vi "Call Function.vi"(7 "Function Name":string, 8 "Error In":errorcluster, 11 "OPI Ref":refnum<data-value>) -> (0 "Error Out":errorcluster, 3 "OPI Ref":refnum<data-value>)   [LabVIEW 2016, in "OPI.lvclass"]
doc: "Call the python function with predefined arguments. The <b>return value</b> and <b>exception information</b> from the function execution will be captured by the OPI. \n\nThe wired function name should be only the name of the function, <b>without</b> parentheses or arguments.\n\nRead return value with <b>Get Return</b>. The exception will be passed into the error cluster output.\n\n<b>Important</b> - the methods called by OPI should not have infinite loops or other mechanisms blocking execution. This can cause a timeout on the OPI."
uses:
  OPI.lvclass
  OPI.lvclass/OPI.ctl
  <vilib>/Utility/error.llb/Error Cluster From Error Code.vi
  <vilib>/ErrorRing/Error Ring.xnode
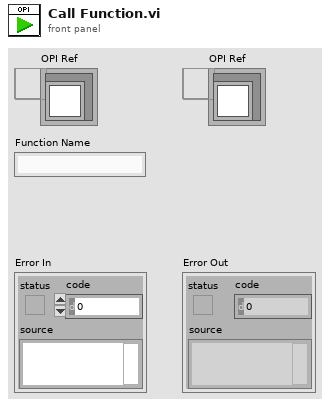
[diagram p1: front panel]
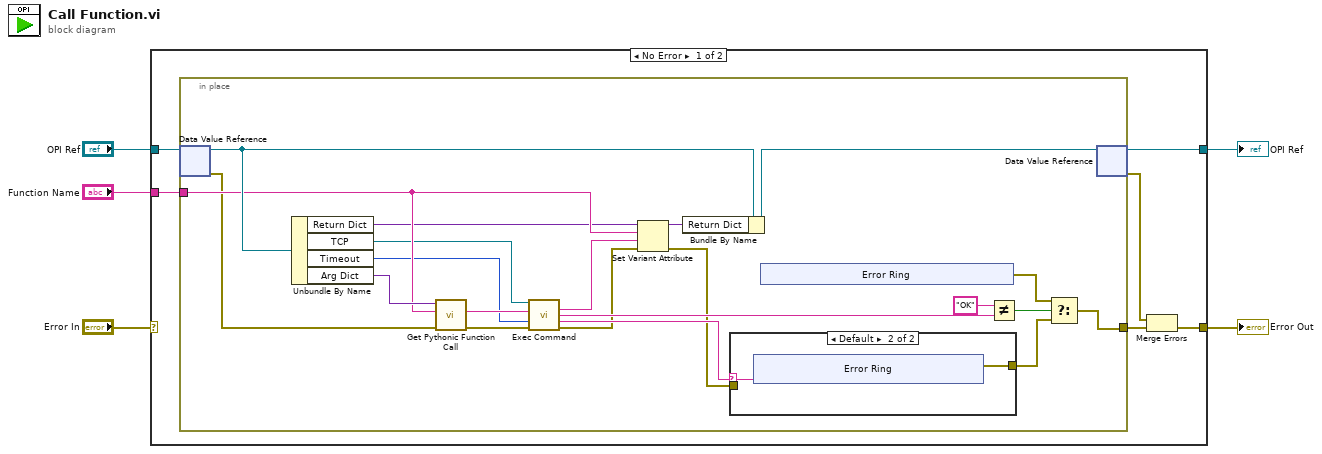
[diagram p0: block diagram]
diagram:
  n1 = case shown="No Error" "Error In" {
    selector: "Error In" -> [_ w48]
    tunnel: [w8 w48] -> w1
    tunnel: "OPI Ref" -> [w11 w49]
    tunnel: [w10 w49] -> w4
    tunnel: "Function Name" -> [w6 _]
    frame No Error {
      n2 = in-place {
        in-place-border: [w28] -> w9
        in-place-border: w6 -> [w18]
        n3 = in-place-dvr #1(w11) -> (w27:refnum<class "OPI.lvclass">, w12:errorcluster)
        n4 = Unbundle By Name(w27) -> ("Return Dict"=w15:variant, "TCP"=w14:refnum<k5>, "Timeout"=w13:i32, "Arg Dict"=w19:variant)
        n5 = call "Get Pythonic Function Call.vi"("Error In"=w12, "Function Name"=w18, "Arg Dict"=w19) -> ("Error Out"=w17:errorcluster, "Function Call"=w16:string)  [unwired: 7 in]
        n6 = call "Exec Command.vi"("TCP In"=w14, "Function Name"=w16, "Timeout"=w13, "Error In"=w17) -> ("Return Value"=w22:string, "OK Ack"=w23:string, "Exception"=w24:string, "Error Out"=w21:errorcluster)  [unwired: 7 in, 1 out]
        n7 = Set Variant Attribute(Variant=w15, name=w18, value=w22, error in=w21) -> (Variant out=w25:variant, error out=w20:errorcluster)  [unwired: 1 out]
        n8 = Bundle By Name(cluster=w27, "Return Dict"=w25) -> (w26:refnum<class "OPI.lvclass">)
        n9 = case shown="Default" w24 {
          selector: w24 -> [_ w40]
          tunnel: [w38 w39] -> w29
          tunnel: w20 -> [w38 _]
          frame "None" {
          }
          frame Default {
            n10 = xnode "Error Ring"("parameter 0"=w40) -> ("error out"=w39:errorcluster)
          }
        }
        n11 = xnode "Error Ring"() -> ("error out"=w30:errorcluster)
        n12 = Not Equal?(x="OK", y=w23) -> (x != y?=w31:bool)
        n13 = Select(t=w30, s=w31, f=w29) -> (s? t:f=w28:errorcluster)
        n14 = in-place-dvr #1(w26) -> (w10:refnum<data-value>, w7:errorcluster)
      }
      n15 = Merge Errors(w7, w9) -> (w8:errorcluster)
    }
    frame Error {
    }
  }
  "Error Out" <- w1
  "OPI Ref" <- w4
